vi "NI_Stop Program and Reset Pos.vi"(8 "return to start":bool, 10 "Program ID":u8 format="%.0x", 11 "Motion Settings In":T1={"No Motion?"=FALSE, "Motion System"=enum."MM3000", "Motion Bd ID"=0, "Motion Profile"="", "# Axis"=0, "Reverse Z axis?"=FALSE, "SMAC Axis"=0, "scan pair"=enum."y-(x) scan", "RT fps"=0.0, "Steps per mm"=[], "Motor Parameters"={"velocity ct/s"=[], "accel ct/s^2"=[]}, "One Way Scan"=FALSE, "Reverse One Way Scan"=FALSE, "Global Position (mm)"=[], "Plane"=0, "Distance between\nscan lines (um)"=0.0, "Distance between\nscan planes (um)"=0.0, "number of scan planes"=0, "Total steps in line"=0, "Xtra plane\ndistance  (um)"=0, "Xtra planes "=0, "Add Axis"=FALSE, "overshoot cts"=0, "BKPT Shift"=0, "Scan Start Time (ms)"=0, "ESP VISA"="", "3rd Axis"=1, "GL Ref Out"=refnum, "Galil Address"=""} {"3rd Axis" items=["x", "y", "z", "w"]; "Xtra planes" min=1; "Xtra plane\ndistance  (um)" min=0; "Distance between\nscan planes (um)" format="%.2f"; "Distance between\nscan lines (um)" format="%.2f"; "SMAC Axis" items=["None"=0, "Axis 1"=1, "Axis 2"=2, "Axis 3"=3, "Axis 4"=4, "Axis 5"=5, "Axis 6"=6, "Axis 7"=7, "Axis 8"=8, "Vector Space 1"=17, "Vector Space 2"=18, "Vector Space 3"=19, "Vector Space 4"=20]; "Motion Bd ID" min=1 max=32 step=1}) -> (3 "Motion Settings":T1={"No Motion?"=FALSE, "Motion System"=enum."NI 735x", "Motion Bd ID"=1, "Motion Profile"="SMAC1", "# Axis"=1, "Reverse Z axis?"=TRUE, "SMAC Axis"=0, "scan pair"=enum."y-(x) scan", "RT fps"=6.0, "Steps per mm"=[1000, 1000, 1000, 1000], "Motor Parameters"={"velocity ct/s"=[10000.0, 10000.0, 10000.0, 50000.0], "accel ct/s^2"=[50000.0, 50000.0, 50000.0, 200000.0]}, "One Way Scan"=FALSE, "Reverse One Way Scan"=FALSE, "Global Position (mm)"=[], "Plane"=0, "Distance between\nscan lines (um)"=0.0, "Distance between\nscan planes (um)"=0.0, "number of scan planes"=1, "Total steps in line"=0, "Xtra plane\ndistance  (um)"=100, "Xtra planes "=1, "Add Axis"=FALSE, "overshoot cts"=200, "BKPT Shift"=0, "Scan Start Time (ms)"=0, "ESP VISA"="GPIB::1::INSTR", "3rd Axis"=1, "GL Ref Out"=refnum, "Galil Address"=""} {"3rd Axis" items=["x", "y", "z", "w"]; "Xtra planes" min=1; "Xtra plane\ndistance  (um)" min=0; "Distance between\nscan planes (um)" format="%.2f"; "Distance between\nscan lines (um)" format="%.2f"; "SMAC Axis" items=["None"=0, "Axis 1"=1, "Axis 2"=2, "Axis 3"=3, "Axis 4"=4, "Axis 5"=5, "Axis 6"=6, "Axis 7"=7, "Axis 8"=8, "Vector Space 1"=17, "Vector Space 2"=18, "Vector Space 3"=19, "Vector Space 4"=20]; "Motion Bd ID" min=1 max=32 step=1})   [LabVIEW 2022 SP3]
uses:
  -NI_MotionRoutines/MotionParameters.ctl
  -NI_MotionRoutines/MotionSys.ctl
  -MotionRoutines/ScanAxis.ctl
  -MotionRoutines/3rdAxis.ctl
  Galil/Command Menu.ctl
  <instrlib>/Newport ESP301/Newport ESP301.lvlib
  <vilib>/Motion/FlexMotion/FunctionsVIs/Trajectory.llb/Load Acceleration/Deceleration.flx
panel:
  # "1-D and 2-D B scan settings"
  # "1-D and 2-D B scan settings"
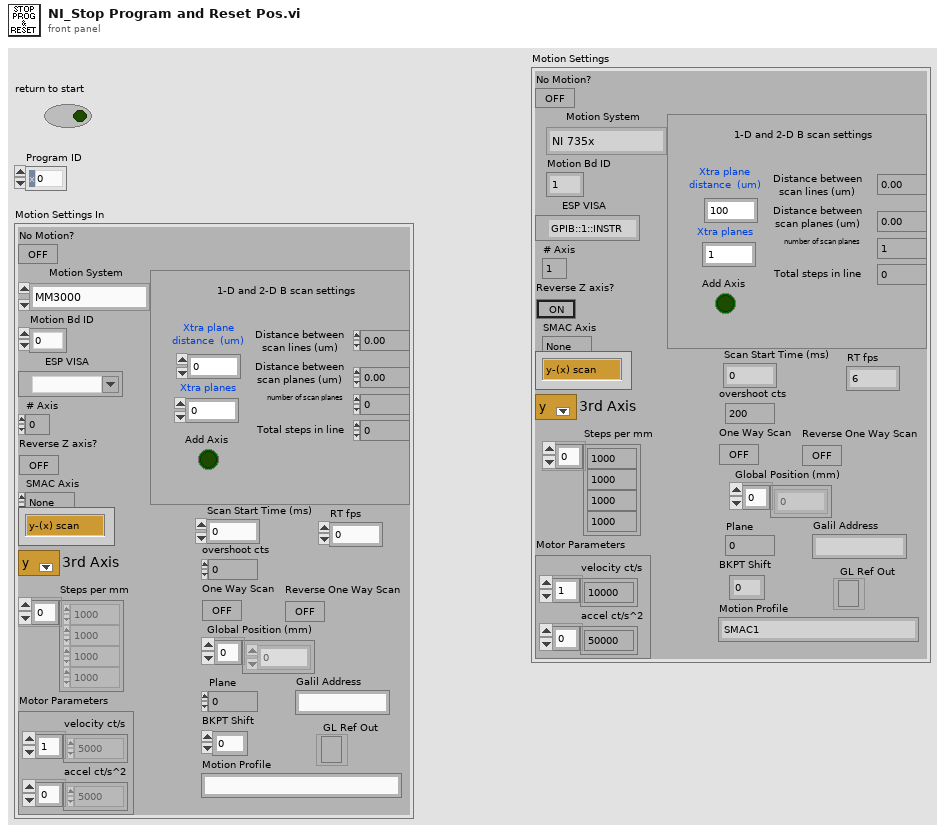
[diagram p1: front panel]
types:
  T1 = typedef "MotionParameters.ctl" = cluster{"No Motion?":bool, "Motion System":T2, "Motion Bd ID":u8, "Motion Profile":string, "# Axis":i8, "Reverse Z axis?":bool, "SMAC Axis":u16, "scan pair":T3, "RT fps":sgl, "Steps per mm":i32[], "Motor Parameters":cluster{"velocity ct/s":dbl[], "accel ct/s^2":dbl[]}, "One Way Scan":bool, "Reverse One Way Scan":bool, "Global Position (mm)":dbl[], "Plane":i32, "Distance between\nscan lines (um)":sgl, "Distance between\nscan planes (um)":sgl, "number of scan planes":i32, "Total steps in line":i32, "Xtra plane\ndistance  (um)":i32, "Xtra planes ":i32, "Add Axis":bool, "overshoot cts":i32, "BKPT Shift":i32, "Scan Start Time (ms)":u32, "ESP VISA":refnum<visa-resource-name>, "3rd Axis":T4, "GL Ref Out":refnum<k7>, "Galil Address":string}
  T2 = typedef "MotionSys.ctl" = enum16{"MM3000", "NI 735x", "Newport ESP", "No Motion Card", "Galil"}
  T3 = typedef "ScanAxis.ctl" = enum16{"y-(x) scan", "x-(y) scan", "z-(x) scan", "z-(y) scan", "y-(z) scan", "x-(z) scan", "w-(x) scan", "w-(y) scan", "w-(z) scan", "x-(w) scan", "y-(w) scan", "z-(w) scan"}
  T4 = typedef "3rdAxis.ctl" = u16
  T5 = typedef "Command Menu.ctl" = enum16{"CommandPassThrough", "Abort Motion", "Define Pos", "Velocity", "Acceleration", "Deceleration", "Position Rel", "Postion Abs", "Begin Move", "After Move", "Home", "KI", "KD", "KP", "IL", "Config I/O", "Set Bit", "Clear Bit", "Motor Off", "Moto On", "Status", "Execute", "Halt Execute", "HX Status", "Tell Velocity", "Check Motion", "BreakPoint", "Tell Position", "Current Code Line", "Tell Switches", "OC Force On", "OC Off", "Pos Soft Limit", "Rev Soft Limit"}
  T6 = typedef "Resource Out.flx" = u8
  T7 = typedef "Bd Id Out" = u8
  T8 = typedef "Resource Out (Enum).flx" = u16
  T9 = typedef "GL Axis Control.ctl" = u16
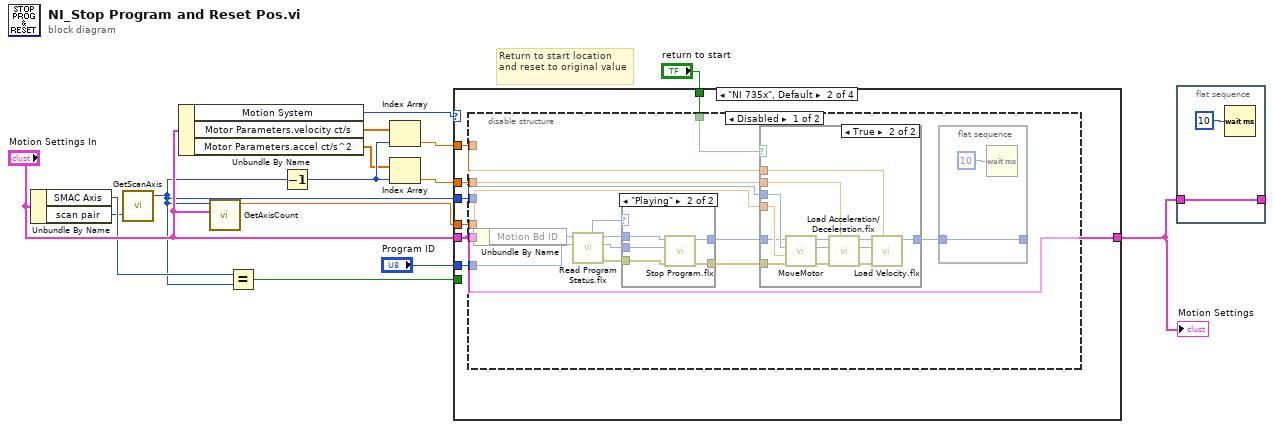
[diagram p0: block diagram]
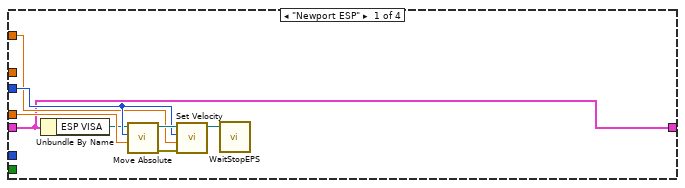
[diagram p2: hidden frame]
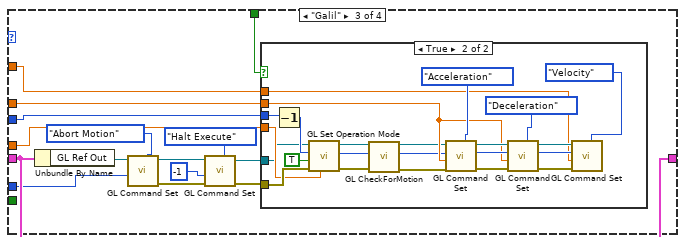
[diagram p6: hidden frame]
diagram:
  # "Return to start location and reset to original value"
  n1 = Unbundle By Name("Motion Settings In") -> ("SMAC Axis"=w6:u16, "scan pair"=w5:T3)
  n2 = call "GetScanAxis.vi"("scan pair"=w5) -> ("Axis 1"=w3:i32)  [unwired: 1 in, 2 out]
  n3 = Unbundle By Name("Motion Settings In") -> ("Motion System"=w15:T2, "Motor Parameters.velocity ct/s"=w8:dbl[], "Motor Parameters.accel ct/s^2"=w9:dbl[])
  n4 = call "GetAxisCount.vi"("Motion Settings"="Motion Settings In", "Scan Axis"=w3) -> ("Counts"=w13:dbl)  [unwired: 9 in]
  n5 = Equal?(x=w6, y=w3) -> (x = y?=w4:bool)
  n6 = Decrement(x=w3) -> (x-1=w10:i32)
  n7 = Index Array(array=w8, index=w10) -> (element=w11:dbl)
  n8 = Index Array(array=w9, index=w10) -> (element=w12:dbl)
  n9 = case shown="\"NI 735x\", Default" w15 {
    tunnel: w3 -> [w20 w30 w83 _]
    tunnel: "Program ID" -> [_ w26 w77 _]
    tunnel: w13 -> [w19 w29 w82 _]
    tunnel: w4 -> [_ _ _ _]
    tunnel: w11 -> [w18 w28 w81 _]
    tunnel: w12 -> [_ w27 w80 _]
    tunnel: "Motion Settings In" -> [w16 w25 w79 w107]
    tunnel: [w16 w25 w79 w107] -> w1
    tunnel: "return to start" -> [_ w24 w75 _]
    frame "Newport ESP" {
      n10 = Unbundle By Name(w16) -> ("ESP VISA"=w17:refnum<visa-resource-name>)
      n11 = call <instrlib>:"Move Absolute.vi"("Position (0 units)"=w19, "Axis (1)"=w20, "VISA resource name"=w17) -> ("error out"=w23:errorcluster, "VISA resource name out"=w21:refnum<visa-resource-name>)  [unwired: 3 in]
      n12 = call <instrlib>:"Set Velocity.vi"("error in (no error)"=w23, "Velocity (units/s)"=w18, "Axis (1)"=w20, "VISA resource name"=w21) -> ("VISA resource name out"=w22:refnum<visa-resource-name>)  [unwired: 2 in, 1 out]
      n13 = call "WaitStopEPS.vi"("VISA resource name"=w22) -> ()  [unwired: 2 in, 3 out]
    }
    frame "NI 735x", Default {
      n14 = disable-structure shown="Disabled" {
        disable-tunnel: w30 -> [w45 _]
        disable-tunnel: w29 -> [w44 _]
        disable-tunnel: w28 -> [w41 _]
        disable-tunnel: w27 -> [w40 _]
        disable-tunnel: w26 -> [w38 _]
        disable-tunnel: w25 -> [w34 _]
        disable-tunnel: w24 -> [w31 _]
        frame Disabled {
          n15 = Unbundle By Name(w34) -> ("Motion Bd ID"=w33:u8)
          n16 = call <vilib>:"Read Program Status.flx"("Program (1)"=w38, "Board Id"=w33) -> ("error out"=w35:errorcluster, "Resource Out"=w37:T6, "Bd Id Out"=w36:T7, "Program Status"=w39:enum16{"Done", "Playing", "Paused", "Storing"})  [unwired: 4 in]
          n17 = case shown="\"Playing\"" w39 {
            tunnel: w36 -> [w63 w68]
            tunnel: w37 -> [_ w67]
            tunnel: [w63 w66] -> w43
            tunnel: [w62 w65] -> w42
            tunnel: w35 -> [w62 w64]
            frame "Done", Default {
            }
            frame "Playing" {
              n18 = call <vilib>:"Stop Program.flx"("error in (no error)"=w64, "Program (1)"=w67, "Board ID"=w68) -> ("error out"=w65:errorcluster, "Bd ID Out"=w66:T7)  [unwired: 4 out]
            }
          }
          n19 = case shown="True" w31 {
            tunnel: w45 -> [_ w54]
            tunnel: w44 -> [_ w59]
            tunnel: w43 -> [w46 w53]
            tunnel: w42 -> [_ w52]
            tunnel: [w46 w58] -> w32
            tunnel: w41 -> [_ w48]
            tunnel: w40 -> [_ w47]
            frame False {
            }
            frame True {
              n20 = call "MoveMotor.vi"("error in (no error)"=w52, "Target Position (0)"=w59, "Axis or Vector Space"=w54, "Motion Bd ID"=w53) -> ("error out"=w50:errorcluster, "Resource Output"=w49:u16, "Bd ID Out"=w51:u8)  [unwired: 5 in]
              n21 = call "Load Acceleration/Deceleration.flx"("Acceleration (100000)"=w47, "error in (no error)"=w50, "Axis or Vector Space"=w49, "Board ID"=w51) -> ("error out"=w57:errorcluster, "Resource Output"=w55:T8, "Bd ID Out"=w56:T7)  [unwired: 1 in, 2 out]
              n22 = call <vilib>:"Load Velocity.flx"("Velocity (10000)"=w48, "error in (no error)"=w57, "Axis or Vector Space"=w55, "Board ID"=w56) -> ("Bd ID Out"=w58:T7)  [unwired: 5 out]
            }
          }
          n23 = flat-sequence {
            tunnel: w32 -> [w60]
            tunnel: [w60] -> _
            frame #0 {
              n24 = Wait (ms)(milliseconds to wait=u32 10) -> ()  [unwired: 1 out]
            }
          }
        }
        frame Enabled {
        }
      }
    }
    frame "Galil" {
      n25 = Unbundle By Name(w79) -> ("GL Ref Out"=w78:refnum<k7>)
      n26 = call "GL Command Set.vi"("Command"=Command_Menu."Abort Motion", "Value"=w77, "Galil.IGalil"=w78) -> ("error out"=w74:errorcluster, "ref out"=w71:refnum<k7>)  [unwired: 4 in, 3 out]
      n27 = call "GL Command Set.vi"("Command"=Command_Menu."Halt Execute", "error in (no error)"=w74, "Value"=-1, "Galil.IGalil"=w71) -> ("error out"=w73:errorcluster, "ref out"=w72:refnum<k7>)  [unwired: 3 in, 3 out]
      n28 = case shown="True" w75 {
        tunnel: w83 -> [_ w93]
        tunnel: w82 -> [_ w94]
        tunnel: w72 -> [_ w86]
        tunnel: w73 -> [_ w95]
        tunnel: w81 -> [_ w97]
        tunnel: w80 -> [_ w96]
        frame False {
        }
        frame True {
          n29 = Decrement(x=w93) -> (x-1=w92:i32)
          n30 = call "GL Set Operation Mode.vi"("position cts (abs/rel)"=w94, "error in (no error)"=w95, "Start Now?"=TRUE, "Axis"=w92, "Galil.IGalil"=w86) -> ("error out"=w90:errorcluster, "Axis Out Output"=w88:T9, "Galil Out"=w87:refnum<k7>)  [unwired: 4 in]
          n31 = call "GL CheckForMotion.vi"("error in"=w90, "Axis"=w88, "Refnum in"=w87) -> ("error out"=w89:errorcluster, "Axis out"=w84:T9, "Refnum out"=w85:refnum<k7>)  [unwired: 6 in]
          n32 = call "GL Command Set.vi"("Command"=Command_Menu."Acceleration", "error in (no error)"=w89, "Value"=w96, "Axis"=w84, "Galil.IGalil"=w85) -> ("error out"=w104:errorcluster, "Axis Out"=w106:T9, "ref out"=w101:refnum<k7>)  [unwired: 2 in, 2 out]
          n33 = call "GL Command Set.vi"("Command"=Command_Menu."Deceleration", "error in (no error)"=w104, "Value"=w96, "Axis"=w106, "Galil.IGalil"=w101) -> ("error out"=w103:errorcluster, "Axis Out"=w105:T9, "ref out"=w102:refnum<k7>)  [unwired: 2 in, 2 out]
          n34 = call "GL Command Set.vi"("Command"=Command_Menu."Velocity", "error in (no error)"=w103, "Value"=w97, "Axis"=w105, "Galil.IGalil"=w102) -> ()  [unwired: 2 in, 5 out]
        }
      }
    }
    frame "No Motion Card" {
    }
  }
  "Motion Settings" <- w1
  n35 = flat-sequence {
    tunnel: w1 -> [w108]
    tunnel: [w108] -> _
    frame #0 {
      n36 = Wait (ms)(milliseconds to wait=u32 10) -> ()  [unwired: 1 out]
    }
  }
